vi "Var_señales_G3.vi"() -> ()   [LabVIEW 2018]
panel:
  in  "Var_V_G3":sgl
  in  "Var_Frec_G3":sgl
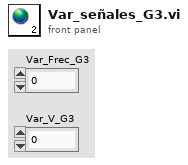
[diagram p1: front panel]
diagram:
